vi "Test Executive.vi"(11 "Module Config":T30={"Name"="Test Executive", "Parent Q"=refnum, "Is Child?"=FALSE, "Index"=0, "Dirs"={"Root"=path "C:/MTE", "Config"=path "C:/MTE/Config", "Logs"=path "C:/MTE/Logs", "Reports"=path "C:/ATE/Reports", "App Data"=path "C:/ProgramData/Test Executive"}, "Simulate"=FALSE, "SimCtrl"=refnum}) -> ()   [LabVIEW 2018] (continued)
              tunnel: [w876] -> w869
              stop <- w876 stop-if-true
              n424 = Unbundle By Name(w880) -> ("Path"=w879:path, "Name"=w878:string)
              n425 = Equal?(x=w878, y=w877) -> (x = y?=w876:bool)
            }
            n426 = case shown="True" w869 {
              tunnel: w870 -> [_ w875]
              tunnel: [_ w874] -> _
              frame False {
              }
              frame True {
                n427 = call <vilib>:"File.Open File or Folder.vi"("Path"=w875) -> ("Error Out"=w874:errorcluster)  [unwired: 10 in]
              }
            }
          }
          frame "Config - Set Test Exec Cfg" {
            n428 = call "TestExec.Configure Test Executive Station Read and Dialog.vi"("Dialog"=TRUE, "TE Config Folder"=path "C:/MTE/Test Executive/Config" ("Path")) -> ("Changed"=w881:bool)  [unwired: 8 in, 1 out]
            n429 = case shown="True" w881 {
              frame False {
              }
              frame True {
                n430 = One Button Dialog(message="Close then relaunch Test Executive for changes to take effect.") -> ()  [unwired: 1 in, 1 out]
              }
            }
          }
          frame "Config - Set Local Station Cfg" {
            n431 = Unbundle By Name(w894) -> ("Cfg.Dirs.Config"=w889:path)
            n432 = Build Path(base path=w889, name or relative path="Local Station.ini") -> (appended path=w888:path)
            n433 = call "TestExec.Configure Local Station ID Read and Dialog.vi"("Dialog"=TRUE, "Config File"=w888) -> ("Changed"=w893:bool, "Station Out"=w890:T4)  [unwired: 8 in]
            n434 = case shown="True" w893 {
              tunnel: w891 -> [w896 w903]
              tunnel: [w896 w902] -> w892
              tunnel: w890 -> [_ w897]
              frame False {
              }
              frame True {
                n435 = Unbundle By Name(w897) -> ("Name"=w901:string, "PN"=w900:string, "SN"=w899:string, "Location"=w898:string)
                n436 = local write "Station"(w897) -> ()
                n437 = Bundle By Name(cluster=w903, "RptHdr.Station.Name"=w901, "RptHdr.Station.PN"=w900, "RptHdr.Station.SN"=w899, "RptHdr.Station.Location"=w898) -> (w902:T73)
              }
            }
          }
          frame "Config - Set File Sync" {
            w925 = T74 -5201 items=["No Error"=0, "Abort"=-2, "Misc"=-5000, "Fixture Error"=-5100, "File IO - General"=-5200, "FIle IO - Config Error"=-5201, "Instrument - General"=-5300, "Instrument - Serial Com"=-5301, "Instrument - Camera"=-5302, "Instrument - PS"=-5303, "Instrument - Oscilloscope"=-5304, "Instrument - Function Gen"=-5305, "Instrument - Load"=-5306, "Instrument - Meter"=-5307, "Instrument - Power Control"=-5308, "Instrument - Motion"=-5309, "Instrument - RF"=-5310, "System Exe"=-5400, "Image Processing"=-5500, "Communication"=-5600, "Script - Syntax Error"=-6000, "Script - Invalid Name or Param"=-6100, "Script - Timeout"=-6200, "Invalid Data"=-6300, "FW Update Error"=-6500] ("Std Code")
            # "If master was edited, copy to local"
            n438 = Variant To Data(type=FALSE, Variant=w929) -> (data=w926:bool, error out=w927:errorcluster)  [unwired: 1 in]
            n439 = flat-sequence {
              tunnel: [errorcluster {"status"=FALSE, "code"=0, "source"=""} ("error constant")] -> w920
              frame #0 {
                n440 = local write "FileSyncActive"(TRUE ("FileSyncActive")) -> ()
              }
            }
            n441 = case shown="No Error" w927 {
              tunnel: w926 -> [w958 _]
              tunnel: [w958 _] -> w915
              frame No Error {
              }
              frame Error {
              }
            }
            n442 = Unbundle By Name(w934) -> ("Cfg.Dirs.Config"=w922:path)
            n443 = Unbundle By Name(w916) -> ("Sync"=w935:refnum<class "File.Sync.lvclass">)
            n444 = Unbundle By Name(w916) -> ("CfgFilePaths.WorkingCfg"=w914:path)
            n445 = Build Path(base path=w922, name or relative path="File Sync Config.csv") -> (appended path=w910:path)
            n446 = local read "Force Sync Now"() -> (w904:bool)
            n447 = call "TestExec.Configure Select Master File Sync Config File.vi"("Dialog"=w915, "File Sync Local"=w910, "Working Config"=w914) -> ("Is Master"=w913:bool, "File Sync File"=w911:path)  [unwired: 7 in]
            n448 = call-dynamic "FileSync.Read Config.vi"("error in (no error)"=w920, "Dialog"=w915, "Config File"=w911, "File.Sync in"=w935) -> ("error out"=w919:errorcluster, "SyncItems"=w908:T14[], "Saved"=w912:bool, "File.Sync out"=w932:refnum<class "File.Sync.lvclass">)  [unwired: 4 in]
            n449 = Or(x="Enable File Sync", y=w904) -> (x .or. y?=w907:bool)
            n450 = Bundle By Name(cluster=w916, "Lists.FileSyncMaster"=w911) -> (w917:T73)
            n451 = And(x=w913, y=w912) -> (x .and. y?=w909:bool)
            n452 = case shown="True" w907 {
              tunnel: w932 -> [w937 w952]
              tunnel: [w937 w950] -> w931
              tunnel: [w938 w949] -> w930
              tunnel: w919 -> [w936 w946]
              tunnel: [w936 w942] -> w918
              tunnel: w908 -> [w938 _]
              tunnel: [_ FALSE] -> w905
              frame False {
              }
              frame True {
                n453 = control-ref of="Status"() -> (w948:refnum<vi>)
                n454 = local read "SyncType"() -> (w940:bool)
                n455 = call "String.Notification Message - Set Text Box State.vi"("error in (no error)"=w946, "Message"="Syncing Config Files, Please Wait.", "TxtBoxRef"=w948) -> ("error out"=w941:errorcluster, "OldColor"=w943:u32, "OldValue"=w944:string, "RefOut"=w945:refnum<vi>)  [unwired: 5 in]
                n456 = call-dynamic "FileSync.Update Sync.vi"("error in (no error)"=w941, "Sync Diff(F) or All(T)"=w940, "Normal(F)/Force Sync(T)"=TRUE, "File.Sync in"=w952) -> ("error out"=w942:errorcluster, "Sync Items"=w949:T14[], "File.Sync out"=w950:refnum<class "File.Sync.lvclass">)  [unwired: 3 in, 2 out]
                n457 = call "String.Notification Message - Set Text Box State.vi"("error in (no error)"=w942, "NewColor"=w943, "Message"=w944, "TxtBoxRef"=w945) -> ()  [unwired: 4 in, 4 out]
              }
            }
            "Sync Items" <- w930
            n458 = case shown="True" w909 {
              tunnel: w911 -> [_ w954]
              tunnel: w910 -> [_ w953]
              frame False {
              }
              frame True {
                n459 = call <vilib>:"File.Copy with Overwrite.vi"("Destination"=w953, "Source"=w954) -> ()  [unwired: 7 in, 3 out]
              }
            }
            n460 = flat-sequence {
              tunnel: w918 -> [_]
              frame #0 {
                n461 = local write "FileSyncActive"(FALSE ("FileSyncActive")) -> ()
              }
            }
            n462 = local write "Force Sync Now"(w905) -> ()
            n463 = Bundle By Name(cluster=w917, "Sync"=w931) -> (w933:T73)
            n464 = call "Error.Set-Change Error Info.vi"("Std Code"=w925, "error in"=w918, "Description"="Sync Files. ") -> ("error out"=w923:errorcluster)  [unwired: 8 in]
          }
          frame "Config - Set Reports" {
            w972 = T74 -5201 items=["No Error"=0, "Abort"=-2, "Misc"=-5000, "Fixture Error"=-5100, "File IO - General"=-5200, "FIle IO - Config Error"=-5201, "Instrument - General"=-5300, "Instrument - Serial Com"=-5301, "Instrument - Camera"=-5302, "Instrument - PS"=-5303, "Instrument - Oscilloscope"=-5304, "Instrument - Function Gen"=-5305, "Instrument - Load"=-5306, "Instrument - Meter"=-5307, "Instrument - Power Control"=-5308, "Instrument - Motion"=-5309, "Instrument - RF"=-5310, "System Exe"=-5400, "Image Processing"=-5500, "Communication"=-5600, "Script - Syntax Error"=-6000, "Script - Invalid Name or Param"=-6100, "Script - Timeout"=-6200, "Invalid Data"=-6300, "FW Update Error"=-6500] ("Std Code")
            n465 = Variant To Data(type=FALSE, Variant=w976) -> (data=w973:bool, error out=w974:errorcluster)  [unwired: 1 in]
            n466 = Unbundle By Name(w978) -> ("Cfg.Dirs.Config"=w966:path)
            n467 = case shown="No Error" w974 {
              tunnel: w973 -> [w979 _]
              tunnel: [w979 _] -> w964
              frame No Error {
              }
              frame Error {
              }
            }
            n468 = Unbundle By Name(w963) -> ("RptCfg"=w962:T17[])
            n469 = Build Path(base path=w966, name or relative path="Reports Config.csv") -> (appended path=w960:path)
            n470 = call "Reports.Report Config - Read.vi"("Config File"=w960, "Dialog"=w964, "Report Config In"=w962) -> ("error out"=w961:errorcluster, "Report Config Out"=w959:T17[])  [unwired: 7 in]
            "Report Config" <- w959
            n471 = Array Size(array=w959) -> (size(s)=w969:i32)
            n472 = Bundle By Name(cluster=w963, "RptCfg"=w959) -> (w977:T73)
            n473 = Initialize Array(cluster{"Open":bool} {"Open"=FALSE} ("Item"), w969) -> (w967:cluster{"Open":bool}[])
            n474 = local write "Open RprFldr"(w967) -> ()
            n475 = call "Error.Set-Change Error Info.vi"("Std Code"=w972, "error in"=w961, "Description"="Report file config.") -> ("error out"=w970:errorcluster)  [unwired: 8 in]
          }
          frame "Config - Mode Manager" {
            n476 = Unbundle By Name(w980) -> ("CfgFilePaths.ModeCfg"=w981:path)
            n477 = call "ModeMgr.Mode Setup Dialog.vi"("Mode Config File"=w981) -> ()  [unwired: 11 in]
          }
          frame "DisableResults" {
            # "DisableResults(1 or 0) \n    By default at each equence start results are enabled\n    1 == this sequence will not generate a report file\n    0 == this sequence will generate a report file"
            n478 = Variant To Data(type=string[] [], Variant=w992) -> (data=w986:string[], error out=w988:errorcluster)  [unwired: 1 in]
            n479 = Index Array(array=w986) -> (element=w985:string)  [unwired: 1 in]
            n480 = Equal?(x=w985, y="1") -> (x = y?=w983:bool)
            n481 = Bundle By Name(cluster=w990, "DisableResults"=w983) -> (w993:T73)
            n482 = case shown="Error" w988 {
              selector: w988 -> [_ w1000]
              tunnel: w987 -> [_ w997]
              tunnel: [_ w995] -> w989
              frame No Error {
              }
              frame Error {
                n483 = Format Into String(format string="Invalid Data to task %s. Expected 1D string.", w997) -> (resulting string=w996:string)  [unwired: 2 in, 1 out]
                n484 = call "Error.Set-Change Error Info.vi"("error in"=w1000, "Description"=w996, "Cust Code(0 = no change)"=-5500 ("Code(0 = no change)")) -> ("error out"=w995:errorcluster)  [unwired: 8 in]
              }
            }
          }
          frame "Get Released SW Files" {
            w1012 = T74 -5201 items=["No Error"=0, "Abort"=-2, "Misc"=-5000, "Fixture Error"=-5100, "File IO - General"=-5200, "FIle IO - Config Error"=-5201, "Instrument - General"=-5300, "Instrument - Serial Com"=-5301, "Instrument - Camera"=-5302, "Instrument - PS"=-5303, "Instrument - Oscilloscope"=-5304, "Instrument - Function Gen"=-5305, "Instrument - Load"=-5306, "Instrument - Meter"=-5307, "Instrument - Power Control"=-5308, "Instrument - Motion"=-5309, "Instrument - RF"=-5310, "System Exe"=-5400, "Image Processing"=-5500, "Communication"=-5600, "Script - Syntax Error"=-6000, "Script - Invalid Name or Param"=-6100, "Script - Timeout"=-6200, "Invalid Data"=-6300, "FW Update Error"=-6500] ("Std Code")
            n485 = for {
              N: 2 -> [_]
              tunnel: w1021 -> [w1036]
              shift-right: [w1034] -> w1023
              shift-left: _ -> [w1035]
              tunnel: w1025 -> [w1033]
              tunnel: [w1032] -> w1020 mode=indexing
              tunnel: [w1031] -> w1019
              i -> [w1037]
              stop <- w1031 stop-if-true
              n486 = case shown="1" w1037 {
                tunnel: w1036 -> [_ _]
                tunnel: [w1045 _] -> w1031
                tunnel: w1035 -> [_ w1054]
                tunnel: [w1042 w1053] -> w1034
                tunnel: w1033 -> [w1044 _]
                tunnel: [_ w1048] -> w1032
                frame 0, Default {
                  n487 = Unbundle By Name(w1044) -> ("CfgFilePaths.WorkingCfg"=w1046:path)
                  n488 = call "TestExec.Config, Get Released SW Folder Info.vi"("Station Info"=w1046) -> ("error out"=w1045:errorcluster, "Rel SW File"=w1043:path, "SW Check En"=w1039:bool, "SW Check Int(s)"=w1040:dbl)  [unwired: 5 in, 2 out]
                  n489 = Bundle By Name(cluster=T42 {"Config Folder"=path "", "Seq Folder"=path "", "Rel SW File"=path "", "SW Check Int(s)"=0.0, "Vers"=variant, "SW Check En"=FALSE}, "Rel SW File"=w1043, "SW Check Int(s)"=w1040, "Vers"=variant, "SW Check En"=w1039) -> (w1042:T42)
                }
                frame 1 {
                  n490 = Unbundle By Name(w1054) -> ("SW Check En"=w1049:bool, "Rel SW File"=w1055:path)
                  n491 = call <vilib>:"File.Check if File or Folder Exists.vi"("Path"=w1055) -> ("error out"=w1056:errorcluster, "Exists"=w1050:bool, "Dup Path"=w1057:path)  [unwired: 6 in, 2 out]
                  n492 = And(x=w1049, y=w1050) -> (x .and. y?=w1051:bool)
                  n493 = case shown="True" w1051 {
                    tunnel: w1057 -> [_ w1061]
                    tunnel: w1056 -> [_ _]
                    tunnel: [_ w1060] -> w1052
                    tunnel: [_ w1059] -> w1048
                    tunnel: [_ w1058] -> w1047
                    frame False {
                    }
                    frame True {
                      n494 = call "TestExec.Config, Get Released SW List.vi"("Path"=w1061) -> ("error out"=w1059:errorcluster, "SW List Array"=w1058:string[][], "SW List"=w1060:variant)  [unwired: 8 in]
                    }
                  }
                  "RelSWVers" <- w1047
                  n495 = Bundle By Name(cluster=w1054, "Vers"=w1052) -> (w1053:T42)
                }
              }
            }
            n496 = Unbundle By Name(w1021) -> ("Cfg.Dirs.Root"=w1017:path)
            n497 = call <vilib>:"Q.Enqueue Task.vi"("Task Name"="Maint - Scheduler", "Q In"=w1007) -> ()  [unwired: 8 in, 2 out]
            n498 = Build Path(base path=w1017, name or relative path="Config") -> (appended path=w1016:path)
            n499 = Unbundle By Name(w1023) -> ("Rel SW File"=w1001:path, "SW Check Int(s)"=w1002:dbl, "Vers"=w1022:variant, "SW Check En"=w1003:bool)
            n500 = Merge Errors(w1020, w1019) -> (w1015:errorcluster)
            n501 = case shown="False" FALSE {
              tunnel: w1016 -> [_ w1030]
              tunnel: w1015 -> [w1027 w1029]
              tunnel: [w1027 w1028] -> w1014
              frame False {
              }
              frame True {
                n502 = call "TestExec.Log SW Sync.vi"("error in (no error)"=w1029, "Folder"=w1030) -> ("error out"=w1028:errorcluster)  [unwired: 9 in]
              }
            }
            n503 = call <vilib>:"High Resolution Relative Seconds.vi"() -> ("relative seconds"=w1008:dbl)
            n504 = Bundle By Name(cluster=T12 {"Check Interval"=0.0, "SW Version List File"=path "", "Enabled"=FALSE} ("SW Check Config"), "Enabled"=w1003, "Check Interval"=w1002, "SW Version List File"=w1001) -> (→"SW Check Config":T12)
            n505 = call "Error.Set-Change Error Info.vi"("Std Code"=w1012, "Append Details"=FALSE, "error in"=w1014, "Description"="Error Reading Released SW Config File.") -> ("error out"=w1013:errorcluster)  [unwired: 7 in]
            n506 = Bundle By Name(cluster=w1025, "Health.LastVerListCk"=w1008, "CfgFilePaths.Rel_SW"=w1001, "Health.VerCkInterval"=w1002, "SW_Vers"=w1022, "Health.SW Check En"=w1003) -> (w1026:T73)
          }
          frame "Init Temp Dir" {
            n507 = Unbundle By Name(w1070) -> ("Cfg.Dirs.Root"=w1069:path)
            n508 = Build Path(base path=w1069, name or relative path="Data") -> (appended path=w1067:path)
            n509 = call <vilib>:"File.Create Folder if Does Not Exist.vi"("Path"=w1067) -> ("Dup Path"=w1065:path)  [unwired: 8 in, 2 out]
            n510 = Build Path(base path=w1065, name or relative path="Temp") -> (appended path=w1066:path)
            n511 = call <vilib>:"File.Create Folder if Does Not Exist.vi"("Path"=w1066) -> ("Dup Path"=w1063:path)  [unwired: 8 in, 2 out]
            n512 = Bundle By Name(cluster=w1062, "CfgFilePaths.DataTemp"=w1063) -> (w1071:T73)
          }
          frame "Maint - Scheduler" {
            n513 = local read "Test State"() -> (w1075:enum32{"Idle", "Running", "Completed"})
            n514 = case shown="\"Idle\", \"Completed\"" w1075 {
              tunnel: w1078 -> [w1082 w1088]
              tunnel: w1077 -> [w1080 w1086]
              tunnel: [w1082 w1085] -> w1076
              tunnel: w1074 -> [w1079 _]
              tunnel: [_ w1084] -> w1073
              tunnel: w1072 -> [_ w1083]
              frame Default {
                # "The station is not idle.\nDo nothing.\n\nMust have returned here due to the scheduled check.\nWhen test is idle again, a maint check will occurr again."
                n515 = call <vilib>:"Scheduler.AddTask.vi"("Interval(s)"=60.0, "Task Name"=w1079, "Sched Name"=w1079, "Q In"=w1080) -> ()  [unwired: 6 in, 2 out]
              }
              frame "Idle", "Completed" {
                n516 = while {
                  shift-right: [w1096] -> w1085
                  shift-left: w1088 -> [w1097]
                  shift-right: [w1094] -> _
                  shift-left: "SW" -> [w1095]
                  tunnel: w1086 -> [w1092]
                  shift-right: [w1091] -> w1084
                  shift-left: _ -> [w1090]
                  tunnel: w1083 -> [w1089]
                  stop <- w1093 stop-if-true
                  n517 = case shown="\"SW Ck\"" w1095 {
                    tunnel: w1097 -> [w1102 w1107 w1154 w1168]
                    tunnel: [w1102 w1107 w1158 w1168] -> w1096
                    tunnel: [w1101 w1105 "Done" "Done"] -> w1094
                    tunnel: [_ _ _ TRUE] -> w1093
                    tunnel: w1092 -> [_ w1110 w1160 _]
                    tunnel: [_ _ w1142 w1165] -> w1091
                    tunnel: w1090 -> [_ _ _ w1165]
                    tunnel: w1089 -> [_ _ w1148 _]
                    frame "SW" {
                      n518 = Unbundle By Name(w1102) -> ("Health.SW Check En"=w1098:bool)
                      n519 = Select(t="SW Ck", s=w1098, f="Sync") -> (s? t:f=w1101:string)
                    }
                    frame "SW Ck" {
                      n520 = Unbundle By Name(w1107) -> ("Health.VerCkInterval"=w1115:dbl)
                      n521 = Unbundle By Name(w1107) -> ("Health.LastVerListCk"=w1120:dbl)
                      n522 = Unbundle By Name(w1107) -> ("Health.LastVerCk"=w1121:dbl)
                      n523 = call <vilib>:"High Resolution Relative Seconds.vi"() -> ("relative seconds"=w1122:dbl)
                      n524 = call <vilib>:"High Resolution Relative Seconds.vi"() -> ("relative seconds"=w1119:dbl)
                      n525 = Subtract(x=w1122, y=w1121) -> (x-y=w1117:dbl)
                      n526 = Subtract(x=w1119, y=w1120) -> (x-y=w1116:dbl)
                      n527 = Subtract(x=w1115, y=w1117) -> (x-y=w1113:dbl)
                      n528 = Subtract(x=w1115, y=w1116) -> (x-y=w1111:dbl)
                      n529 = Less Or Equal To 0?(x=w1111) -> (x <= 0?=w1112:bool)
                      n530 = case shown="False" w1112 {
                        tunnel: "Get Released SW Files" -> [w1126 w1128]
                        tunnel: w1110 -> [w1125 w1129]
                        tunnel: w1111 -> [w1124 _]
                        tunnel: [w1123 w1127] -> w1109
                        frame False {
                          n531 = call <vilib>:"Scheduler.AddTask.vi"("Interval(s)"=w1124, "Task Name"=w1126, "Sched Name"=w1126, "Q In"=w1125) -> ("Q Out"=w1123:refnum<queue>)  [unwired: 6 in, 1 out]
                        }
                        frame True {
                          n532 = call <vilib>:"Q.Enqueue Task.vi"("Task Name"=w1128, "Q In"=w1129) -> ("Q Out"=w1127:refnum<queue>)  [unwired: 8 in, 1 out]
                        }
                      }
                      n533 = local read "Enable File Sync"() -> (w1103:bool)
                      n534 = Less Or Equal To 0?(x=w1113) -> (x <= 0?=w1114:bool)
                      n535 = case shown="True" w1114 {
                        tunnel: "Maint - SW Version Check" -> [w1132 w1133]
                        tunnel: w1109 -> [w1131 w1134]
                        tunnel: w1113 -> [w1130 _]
                        frame False {
                          n536 = call <vilib>:"Scheduler.AddTask.vi"("Interval(s)"=w1130, "Task Name"=w1132, "Sched Name"=w1132, "Q In"=w1131) -> ()  [unwired: 6 in, 2 out]
                        }
                        frame True {
                          n537 = call <vilib>:"Q.Enqueue Task.vi"("Task Name"=w1133, "Q In"=w1134) -> ()  [unwired: 8 in, 2 out]
                        }
                      }
                      n538 = Select(t="Sync", s=w1103, f="Done") -> (s? t:f=w1105:string)
                    }
                    frame "Sync" {
                      w1159 = "Maint - Scheduler"
                      n539 = control-ref of="Status"() -> (w1137:refnum<vi>)
                      n540 = property on="FileSyncActive" class="Bool (strict)"("Value"=TRUE ("FileSyncActive")) -> (error out=w1150:errorcluster)  [unwired: 2 in, 1 out]
                      n541 = Unbundle By Name(w1154) -> ("Sync"=w1156:refnum<class "File.Sync.lvclass">)
                      n542 = call "String.Notification Message - Set Text Box State.vi"("Message"="Syncing Config Files, Please Wait.", "TxtBoxRef"=w1137) -> ("OldColor"=w1138:u32, "OldValue"=w1139:string, "RefOut"=w1140:refnum<vi>)  [unwired: 6 in, 1 out]
                      n543 = call-dynamic "FileSync.Update Sync.vi"("error in (no error)"=w1150, "Sync Diff(F) or All(T)"="SyncType", "File.Sync in"=w1156) -> ("error out"=w1142:errorcluster, "Sync Items"=w1151:T14[], "File.Sync out"=w1155:refnum<class "File.Sync.lvclass">, "Next Sync"=w1152:dbl)  [unwired: 4 in, 1 out]
                      n544 = local write "Sync Items"(w1151) -> ()
                      n545 = case shown="Error" w1142 {
                        tunnel: ["File Sync Success" "File Sync Error"] -> w1146
                        frame No Error {
                        }
                        frame Error {
                        }
                      }
                      n546 = call "String.Notification Message - Set Text Box State.vi"("error in (no error)"=w1142, "NewColor"=w1138, "Message"=w1139, "TxtBoxRef"=w1140) -> ("error out"=w1141:errorcluster)  [unwired: 4 in, 3 out]
                      n547 = Bundle By Name(cluster=w1154, "Sync"=w1155) -> (w1153:T73)
                      n548 = Unbundle By Name(w1148) -> ("Log"=w1147:refnum<class "Event Notification.lvclass">)
                      n549 = flat-sequence {
                        tunnel: w1141 -> [_]
                        frame #0 {
                          n550 = property on="FileSyncActive" class="Bool (strict)"("Value"=FALSE ("FileSyncActive")) -> ()  [unwired: 2 in, 2 out]
                        }
                      }
                      n551 = Bundle By Name(cluster=w1153, "Health.Init"=FALSE) -> (w1158:T73)
                      n552 = call <vilib>:"Scheduler.AddTask.vi"("Interval(s)"=w1152, "Task Name"=w1159, "Sched Name"=w1159, "Q In"=w1160) -> ()  [unwired: 6 in, 2 out]
                      n553 = call <vilib>:"Event Notification.Status Message.vi"("Display"=FALSE, "Log"=TRUE, "Level"=Event_Log.Log_Level."Verbose", "Message"=w1146, "Event Notification in"=w1147) -> ()  [unwired: 7 in]
                    }
                    frame "Done", Default {
                    }
                  }
                }
              }
            }
          }
          frame "Maint - SW Version Check" {
            # "TODO: \nAt launch:\n  Need to get version from Sta\n  Get version of all seq and limit at init"
            n554 = Unbundle By Name(w1175) -> ("SW_Vers"=w1177:variant, "RptHdr.Station.SW_Config.SW_Item"=w1178:T31[])  [unwired: 1 out]
            n555 = call <vilib>:"High Resolution Relative Seconds.vi"() -> ("relative seconds"=w1176:dbl)
            n556 = Get Date/Time In Seconds() -> (seconds since 1Jan1904=→"LastVerCkTime":timestamp)
            n557 = Bundle By Name(cluster=w1175, "Health.LastVerCk"=w1176) -> (w1174:T73)
            n558 = call <vilib>:"Q.Enqueue Task.vi"("Task Name"="Maint - Scheduler", "Q In"=w1172) -> ("Q Out"=w1171:refnum<queue>)  [unwired: 8 in, 1 out]
            n559 = for {
              tunnel: w1178 -> [w1190] mode=indexing
              tunnel: w1177 -> [w1191]
              tunnel: w1171 -> [w1188]
              tunnel: [w1184] -> w1169 mode=indexing
              n560 = Unbundle By Name(w1190) -> ("Name"=w1185:string, "PN"=w1182:string, "Version"=w1183:string)
              n561 = Get Variant Attribute(Variant=w1191, name=w1185, default value (empty Variant)="") -> (found=w1180:bool, value=w1186:string)  [unwired: 1 in, 2 out]
              n562 = Not Equal?(x=w1183, y=w1186) -> (x != y?=w1187:bool)
              n563 = And(x=w1180, y=w1187) -> (x .and. y?=w1181:bool)
              n564 = Bundle("Name"=w1185, "PN"=w1182, "Version"=w1183, w1180, w1181) -> (w1184:T75)  [unwired: 1 in]
              n565 = case shown="True" w1181 {
                tunnel: w1188 -> [_ w1200]
                tunnel: w1185 -> [_ w1193]
                tunnel: w1186 -> [_ w1196]
                tunnel: w1183 -> [_ w1194]
                frame False {
                }
                frame True {
                  n566 = Format Into String(format string="SW '%s' is not the released version.  Local ver is '%s' and released ver is '%s'.", w1193, w1194, w1196) -> (resulting string=w1195:string)  [unwired: 2 in, 1 out]
                  n567 = Bundle By Name(cluster=errorcluster {"status"=TRUE, "code"=7000, "source"=""} ("error constant"), "source"=w1195) -> (w1198:errorcluster)
                  n568 = To Variant(anything=TestExec.Health_State_Command."Set Warning" ("Health State Cmd")) -> (Variant=w1204:variant)
                  n569 = To Variant(anything=w1198) -> (Variant=w1201:variant)
                  n570 = call <vilib>:"Q.Enqueue App.vi"("Data2"=w1201, "Top of Q"=TRUE, "Data1"=w1204, "Task Name"="Health Status", "Q In"=w1200) -> ()  [unwired: 5 in, 2 out]
                }
              }
            }
            "Station SW Versions" <- w1169
          }
          frame "Operator - Create Report" {
            # "TODO - Create Report"
            n571 = Unbundle By Name(w1205) -> ()  [unwired: 1 out]
          }
          frame "Operator - Operator Change" {
            n572 = local read "Test Ctrl Tab"() -> (w1211:enum32{"Idle", "Running", "Completed"})
            n573 = call <vilib>:"Trim Whitespace.vi"("string"="Operator") -> ("trimmed string"=w1207:string)  [unwired: 1 in]
            n574 = Bundle By Name(cluster=w1210, "RptHdr.Test Run.Operator"=w1207) -> (w1209:T73)
            n575 = local write "Operator"(w1207) -> ()
            n576 = case shown="\"Idle\"" w1211 {
              tunnel: w1212 -> [_ w1214]
              frame Default {
              }
              frame "Idle" {
                n577 = To Variant(anything="Operator Change" ("Task Name")) -> (Variant=w1216:variant)
                n578 = call <vilib>:"Q.Enqueue Seq.vi"("Data1"=w1216, "Seq Task Name"="Test Idle" ("Task Name"), "Q In"=w1214) -> ()  [unwired: 7 in, 2 out]
              }
            }
          }
          frame "Operator - Set Mode" {
            n579 = Variant To Data(type=FALSE, Variant=w1222) -> (data=w1219:bool, error out=w1220:errorcluster)  [unwired: 1 in]
            n580 = Unbundle By Name(w1231) -> ("ModeMgr"=w1230:refnum<class "Mode Manager.lvclass">)
            n581 = case shown="No Error" w1220 {
              tunnel: w1219 -> [w1232 _]
              tunnel: [w1232 FALSE] -> w1218
              frame No Error {
              }
              frame Error {
              }
            }
            n582 = call "ModeMgr.Set Mode.vi"("Init"=w1218, "ModeMgr In"=w1230) -> ("Settings"=w1225:T76[], "Mode"=w1226:string, "ModeMgr Out"=w1229:refnum<class "Mode Manager.lvclass">, "Changed"=w1223:bool)  [unwired: 5 in, 1 out]
            n583 = case shown="True" w1223 {
              tunnel: w1231 -> [w1234 w1242]
              tunnel: w1229 -> [_ w1248]
              tunnel: [w1234 w1247] -> w1228
              tunnel: w1226 -> [_ w1241]
              tunnel: w1225 -> [_ w1246]
              tunnel: w1224 -> [_ w1244]
              frame False {
              }
              frame True {
                n584 = Unbundle By Name(w1242) -> ("Lists.DisableRouteCk"=w1238:bool)
                n585 = call <vilib>:"Q.Enqueue Task.vi"("Task Name"="Options - Set", "Q In"=w1244) -> ("Q Out"=w1236:refnum<queue>)  [unwired: 8 in, 1 out]
                n586 = call "TestExec.Set Option Controls.vi"("Disable SN Route Ck"=w1238, "TE Opts"=w1246, "TE Opts In"=T20 {"DispDetails"=FALSE, "NotResetSN"=FALSE, "NotValOper"=FALSE, "NotValSN"=FALSE, "DisResults"=FALSE, "StaModule"=FALSE, "EditEQ"=FALSE, "ClrWarn"=FALSE, "ClrErr"=FALSE, "ViewCfg"=FALSE, "SetOpts"=FALSE, "ContOnErr"=FALSE, "ContOnFail"=FALSE, "DisMetrics"=FALSE, "SelSeq"=FALSE, "GenRpt"=FALSE, "DisStartWithSN"=FALSE, "Auto Repeat Seq En"=FALSE, "DataDirEn"=FALSE, "SNRouteCk"=FALSE} ("Opts")) -> ("TE Opts Out"=w1239:T20)  [unwired: 8 in]
                n587 = call <vilib>:"Q.Enqueue Seq.vi"("Seq Task Name"="Test Reset", "Q In"=w1236) -> ()  [unwired: 8 in, 2 out]
                n588 = Unbundle By Name(w1239) -> ("SNRouteCk"=w1237:bool)
                n589 = Equal?(x=w1241, y="Production") -> ()  [unwired: 1 out]
                n590 = local write "TE Opts"(w1239) -> ()
                n591 = Bundle By Name(cluster=w1242, "ModeMgr"=w1248, "RptHdr.Test Run.Mode"=w1241, "Opts"=w1239) -> (w1247:T73)
                n592 = local write "Route Check"(w1237) -> ()
              }
            }
          }
          frame "Operator - Set Result EN" {
            n593 = control-ref of="Result Sel"() -> (w1249:refnum<vi>)
            n594 = Greater Than 0?(x="ReportEn") -> (x > 0?=w1250:bool)
            n595 = call "TestExec.Result Option, Set Enable_Disabel Color.vi"("Result Sel"=w1249) -> ()  [unwired: 11 in]
            n596 = Bundle By Name(cluster=w1255, "Opts.DisResults"=w1250) -> (w1254:T73)
            n597 = local read "TE Opts"() -> (w1253:T20)
            n598 = Bundle By Name(cluster=w1253, "DisResults"=w1250) -> (w1252:T20)
            n599 = local write "TE Opts"(w1252) -> ()
          }
          frame "Operator - SN Change" {
            n600 = local read "Test Ctrl Tab"() -> (w1261:enum32{"Idle", "Running", "Completed"})
            n601 = call <vilib>:"Trim Whitespace.vi"("string"="SN") -> ("trimmed string"=w1257:string)  [unwired: 1 in]
            n602 = local write "SN"(w1257) -> ()
            n603 = Bundle By Name(cluster=w1260, "RptUUT.UUTInfo.SN"=w1257) -> (w1259:T73)
            n604 = case shown="\"Idle\"" w1261 {
              tunnel: w1262 -> [_ w1265]
              frame Default {
              }
              frame "Idle" {
                n605 = To Variant(anything="SN Change") -> (Variant=w1267:variant)
                n606 = call <vilib>:"Q.Enqueue Seq.vi"("Data1"=w1267, "Seq Task Name"="Test Idle" ("Task Name"), "Q In"=w1265) -> ()  [unwired: 7 in, 2 out]
              }
            }
          }
          frame "Operator Comment" {
            w1275 = T39 0 items=["LOG", "PASS", "FAIL", "ERROR"] ("Status")
            w1277 = "Comment"
            n607 = Variant To Data(type="", Variant=w1281) -> (data=w1276:string)  [unwired: 1 in, 1 out]
            n608 = Bundle By Name(cluster=T43 {"Cnt"=0, "Step"="", "Category"="", "Name"="", "Value"="", "Status"=0, "Code"=0, "Desc"="", "Time"=timestamp(0 s since 1904-01-01)} ("Attribute"), "Category"=w1277, "Name"=w1277, "Value"=w1276, "Status"=w1275, "Code"=0, "Desc"="") -> (w1272:T43)
            n609 = Build Array(w1272) -> (w1271:T43[])
            n610 = To Variant(anything=w1271) -> (Variant=w1270:variant)
            n611 = call <vilib>:"Q.Enqueue Task.vi"("Data1"=w1270, "Task Name"="Result - Attributes" ("Desc"), "Q In"=w1268) -> ()  [unwired: 7 in, 2 out]
          }
          frame "Operator YesNo Input" {
            n612 = Variant To Data(type=FALSE, Variant=w1295) -> (data=w1287:bool)  [unwired: 1 in, 1 out]
            n613 = Select(t="Yes", s=w1287, f="No") -> (s? t:f=w1284:string)
            n614 = Unbundle By Name(w1293) -> ("SeqMgr"=w1290:refnum<class "SeqMgr.lvclass">)
            n615 = Build Array("Operator_YesNo_Input", w1284) -> (w1289:string[])
            n616 = Build Array(w1289) -> (w1283:string[][])
            n617 = call <vilib>:"SeqMgr.Variables - Add, Replace.vi"("Name, Value"=w1283, "SeqMgr in"=w1290) -> ("SeqMgr out"=w1291:refnum<class "SeqMgr.lvclass">)  [unwired: 8 in, 1 out]
            n618 = Bundle By Name(cluster=w1293, "SeqMgr"=w1291) -> (w1292:T73)
          }
          frame "Result Comment" {
            n619 = local read "Start Time"() -> (w1299:timestamp)
            n620 = Unbundle By Name(w1304) -> ("RptHdr.Test Run.Comment"=w1321:string)
            n621 = local read "Comment At End"() -> (w1319:bool)
            n622 = Unbundle By Name(w1304) -> ("SeqMgr"=w1305:refnum<class "SeqMgr.lvclass">)
            n623 = Unbundle By Name(w1304) -> ("Lists.CmtPrmpt"=w1320:bool)
            n624 = call <vilib>:"SeqMgr.Variables - Get.vi"("SeqMgr in"=w1305) -> ("Vars"=w1303:variant)  [unwired: 8 in, 2 out]
            n625 = Format Date/Time String(time format string (%c)="%Y%m%d_%H%M%S", seconds (now)=w1299) -> (date/time string=w1297:string)  [unwired: 1 in]
            n626 = call <vilib>:"SeqMgr.Variables, Populate Variable Value Including Array Indices.vi"("String"="UUTDir", "Variables"=w1303) -> ("error out"=w1302:errorcluster, "String Out"=w1298:string)  [unwired: 7 in, 1 out]
            n627 = case shown="False" w1320 {
              tunnel: w1321 -> [_ w1329]
              tunnel: [w1325 w1329] -> w1313
              tunnel: w1319 -> [w1324 _]
              tunnel: "Comment" -> [w1323 _]
              frame False {
                n628 = case shown="False" w1324 {
                  tunnel: [w1326 w1328] -> w1325
                  tunnel: w1323 -> [w1326 w1327]
                  frame False {
                  }
                  frame True {
                    n629 = call "TestExec.Prompt for entering Comment.vi"("Comment"=w1327) -> ("Comment Out"=w1328:string)  [unwired: 10 in]
                  }
                }
              }
              frame True {
                # "Already entered comment"
              }
            }
            n630 = Unbundle By Name(w1306) -> ("Log"=w1310:refnum<class "Event Notification.lvclass">)
            n631 = call <vilib>:"Clear Errors.vi"("error in (no error)"=w1302) -> ()  [unwired: 5 in, 2 out]
            n632 = Format Into String(format string="Test End.  Start Time = \"%s\", UUTDir = \"%s\"", w1297, w1298) -> (resulting string=w1311:string)  [unwired: 2 in, 1 out]
            n633 = call <vilib>:"Event Notification.Status Message.vi"("Log"=TRUE, "Level"=Event_Log.Log_Level."Debug1", "Message"=w1311, "Event Notification in"=w1310) -> ()  [unwired: 8 in]
            n634 = case shown="False" "PersistCmt" {
              tunnel: w1313 -> [_ _]
              frame False {
                n635 = invoke on="Comment" class="Str" method="Reinit To Default"() -> ()  [unwired: 3 in, 3 out]
              }
              frame True {
              }
            }
            n636 = call <vilib>:"Search and Replace Pattern.vi"("string"=w1313, "regular expression (\"\")"="\n", "replace string (\"\")"="| " ("regular expression (\"\")"), "replace all? (F)"=TRUE) -> ("result string"=w1317:string)  [unwired: 1 in, 1 out]
            n637 = Bundle By Name(cluster=w1304, "RptHdr.Test Run.Comment"=w1317) -> (w1322:T73)
          }
          frame "Options - Set" {
            n638 = Bundle By Name(cluster=w1332, "Opts"="TE Opts") -> (w1330:T73)
            n639 = while {
              tunnel: "TE Opts" -> [w1339]
              tunnel: w1333 -> [w1338]
              tunnel: w1332 -> [w1337]
              shift-right: [w1335] -> w1331
              shift-left: w1330 -> [w1336]
              i -> [w1340]
              stop <- w1341 stop-if-true
              n640 = case shown="13" w1340 {
                tunnel: [_ _ _ _ _ _ _ _ _ _ _ _ _ _ TRUE] -> w1341
                tunnel: w1339 -> [w1345 w1359 w1366 w1372 w1378 w1393 w1408 w1424 w1433 w1440 w1447 w1458 w1473 _ _]
                tunnel: w1338 -> [_ w1352 _ _ _ w1389 w1406 _ _ _ _ _ w1469 _ _]
                tunnel: w1337 -> [_ _ _ _ _ w1384 w1403 w1421 _ _ _ w1463 _ w1480 _]
                tunnel: [_ _ _ _ _ _ w1399 _ _ _ _ _ w1467 _ _] -> _
                tunnel: w1336 -> [w1342 w1348 w1363 w1369 w1375 w1381 w1394 w1418 w1431 w1436 w1445 w1455 w1466 w1481 w1487]
                tunnel: [w1342 w1348 w1363 w1369 w1375 w1381 w1394 w1419 w1431 w1436 w1445 w1455 w1466 w1481 w1487] -> w1335
                frame 0 {
                  n641 = Unbundle By Name(w1345) -> ("DispDetails"=w1343:bool)
                  n642 = property on="Test Status Tab" class="TabCtl (strict)"("Tabs Visible?"=w1343) -> (error out=w1344:errorcluster)  [unwired: 2 in, 1 out]
                  n643 = property on="Image Path" class="Path"("Visible"=w1343) -> ()  [unwired: 2 in, 2 out]
                  n644 = case shown="False" w1343 {
                    tunnel: w1344 -> [w1347 _]
                    frame False {
                      n645 = property on="Test Status Tab" class="TabCtl (strict)"(error in=w1347, "Value"=0) -> ()  [unwired: 1 in, 2 out]
                    }
                    frame True {
                    }
                  }
                }
                frame 1 {
                  w1353 = "Show Station Module"
                  n646 = Unbundle By Name(w1359) -> ("StaModule"=w1351:bool)
                  n647 = case shown="False" w1351 {
                    tunnel: [_ TRUE] -> w1350
                    tunnel: [T36."Disabled and Grayed Out" ("Disabled") T36."Enabled" ("Disabled")] -> w1349
                    frame False {
                    }
                    frame True {
                    }
                  }
                  n648 = Unbundle By Name(w1352) -> ("Menu Ref"=w1358:refnum<k9>)
                  n649 = Get Menu Item Info(7:w1353, 11:w1358) -> (0:w1355:errorcluster, 2:w1356:string, 3:w1357:refnum<k9>)  [unwired: 1 in, 4 out]
                  n650 = property on="Show Station Module" class="Bool"("DisabledEnum"=w1349) -> ()  [unwired: 2 in, 2 out]
                  n651 = Set Menu Item Info(7:w1353, 8:w1355, 9:w1350, 10:w1356, 11:w1357) -> (0:w1354:errorcluster)  [unwired: 2 in, 1 out]
                  n652 = call <vilib>:"Clear Errors.vi"("error in (no error)"=w1354) -> ()  [unwired: 5 in, 2 out]
                }
                frame 2 {
                  n653 = Unbundle By Name(w1366) -> ("EditEQ"=w1365:bool)
                  n654 = case shown="False" w1365 {
                    tunnel: [T36."Disabled" ("Disabled") T36."Enabled" ("Disabled")] -> w1364
                    frame False {
                    }
                    frame True {
                    }
                  }
                  n655 = property on="Equipment List" class="Tbl (strict)"("DisabledEnum"=w1364) -> ()  [unwired: 2 in, 2 out]
                }
                frame 3 {
                  n656 = Unbundle By Name(w1372) -> ("ClrWarn"=w1371:bool)
                  n657 = case shown="False" w1371 {
                    tunnel: [T36."Disabled and Grayed Out" ("Disabled") T36."Enabled" ("Disabled")] -> w1370
                    frame False {
                    }
                    frame True {
                    }
                  }
                  n658 = property on="Clear Warnings" class="Bool"("DisabledEnum"=w1370) -> ()  [unwired: 2 in, 2 out]
                }
                frame 4 {
                  n659 = Unbundle By Name(w1378) -> ("ClrErr"=w1377:bool)
                  n660 = case shown="False" w1377 {
                    tunnel: [T36."Disabled and Grayed Out" ("Disabled") T36."Enabled" ("Disabled")] -> w1376
                    frame False {
                    }
                    frame True {
                    }
                  }
                  n661 = property on="Clear Errors" class="Bool"("DisabledEnum"=w1376) -> ()  [unwired: 2 in, 2 out]
                  n662 = property on="Clear Errors and Warnings" class="Bool"("DisabledEnum"=w1376) -> ()  [unwired: 2 in, 2 out]
                  n663 = property on="Test Metrics Reset" class="Bool"("DisabledEnum"=w1376) -> ()  [unwired: 2 in, 2 out]
                  n664 = property on="Test Cycle Cnt Reset" class="Bool"("DisabledEnum"=w1376) -> ()  [unwired: 2 in, 2 out]
                }
                frame 5 {
                  w1390 = "Config" ("menu tag")
                  n665 = Unbundle By Name(w1384) -> ("RptHdr.Test Run.Mode"=w1387:string)
                  n666 = Unbundle By Name(w1393) -> ("ViewCfg"=w1383:bool)
                  n667 = Equal?(x=w1387, y="Engineering") -> (x = y?=w1385:bool)
                  n668 = Or(x=w1383, y=w1385) -> (x .or. y?=w1382:bool)
                  n669 = control-ref of="Funct Tab"() -> (w1392:refnum<vi>)
                  n670 = Unbundle By Name(w1389) -> ("Menu Ref"=w1388:refnum<k9>)
                  n671 = call <vilib>:"CtrlUtil.ShowHide Tab Page.vi"("Show"=w1382, "Tab Name"="Config", "Tab Control"=w1392) -> ()  [unwired: 2 in]
                  n672 = Set Menu Item Info(7:w1390, 9:w1382, 10:w1390, 11:w1388) -> ()  [unwired: 3 in, 2 out]
                }
                frame 6 {
                  n673 = Unbundle By Name(w1403) -> ("RptHdr.Test Run.Mode"=w1405:string)
                  n674 = Unbundle By Name(w1408) -> ("SetOpts"=w1401:bool)
                  n675 = Unbundle By Name(w1406) -> ("Menu Ref"=w1395:refnum<k9>)
                  n676 = Equal?(x=w1405, y="Engineering") -> (x = y?=w1402:bool)
                  n677 = Or(x=w1401, y=w1402) -> (x .or. y?=w1400:bool)
                  n678 = case shown="False" w1400 {
                    tunnel: [T36."Disabled and Grayed Out" ("Disabled") w1416] -> w1398
                    tunnel: [T36."Disabled" ("Disabled") w1416] -> w1407
                    tunnel: [_ TRUE] -> w1397
                    frame False {
                    }
                    frame True {
                      w1416 = T36."Enabled" ("Disabled")
                    }
                  }
                  n679 = property on="Configure Reports" class="Bool"("DisabledEnum"=w1398) -> ()  [unwired: 2 in, 2 out]
                  n680 = property on="Open SW Version File" class="Bool"("DisabledEnum"=w1398) -> ()  [unwired: 2 in, 2 out]
                  n681 = for {
                    tunnel: [w1412] -> w1399
                    tunnel: w1397 -> [w1411]
                    tunnel: string[] ["Test Executive", "Local Station", "File Sync", "Test Reports", "Mode Manager", "Config_Config Folder", "Config_Test Sequence Folder"] -> [w1410] mode=indexing
                    tunnel: w1395 -> [w1409]
                    n682 = call <vilib>:"Menu.Enable Item.vi"("Enable"=w1411, "Tag"=w1410, "Menu Ref"=w1409) -> ("error out"=w1412:errorcluster)  [unwired: 7 in, 1 out]
                  }
                  n683 = property on="Result Sel" class="Ring (strict)"("DisabledEnum"=w1407) -> ()  [unwired: 2 in, 2 out]
                  n684 = property on="TE Opts" class="Clust (strict)"("DisabledEnum"=w1398) -> ()  [unwired: 2 in, 2 out]
                }
                frame 7 {
                  n685 = Unbundle By Name(w1421) -> ("Lists.Default Seq"=w1420:i32)
                  n686 = Unbundle By Name(w1424) -> ("SelSeq"=w1423:bool)
                  n687 = case shown="False" w1423 {
                    tunnel: [T36."Disabled" ("Disabled") T36."Enabled" ("Disabled")] -> w1417
                    tunnel: [u32 0 u32 16860] -> w1422
                    tunnel: w1420 -> [w1425 _]
                    frame False {
                      n688 = To Unsigned Word Integer(number=w1425) -> (unsigned 16bit integer=w1426:u16)
                      n689 = property on="Sequence" class="Ring (strict)"("Value"=w1426) -> ()  [unwired: 2 in, 2 out]
                    }
                    frame True {
                    }
                  }
                  n690 = property on="Sequence" class="Ring (strict)"("DisabledEnum"=w1417, "RingText.TextColor"=w1422) -> ()  [unwired: 2 in, 2 out]
                  n691 = Bundle By Name(cluster=w1418, "PreTestCk.SeqEn"=w1417) -> (w1419:T73)
                }
                frame 8 {
                  n692 = Unbundle By Name(w1433) -> ("GenRpt"=w1432:bool)
                  n693 = case shown="False" w1432 {
                    tunnel: [T36."Disabled and Grayed Out" ("Disabled") T36."Enabled" ("Disabled")] -> _
                    frame False {
                    }
                    frame True {
                    }
                  }
                }
                frame 9 {
                  n694 = Unbundle By Name(w1440) -> ("DisStartWithSN"=w1439:bool)
                  n695 = case shown="True" w1439 {
                    tunnel: [T36."Disabled and Grayed Out" ("Disabled") T36."Enabled" ("Disabled")] -> w1438
                    tunnel: [TRUE w1443] -> w1437
                    frame False {
                    }
                    frame True {
                      n696 = local read "Start with SN Entry"() -> (w1443:bool)
                    }
                  }
                  n697 = local write "Start with SN Entry"(w1437) -> ()
                  n698 = property on="Start with SN Entry" class="Bool (strict)"("DisabledEnum"=w1438) -> ()  [unwired: 2 in, 2 out]
                }
                frame 10 {
                  n699 = Unbundle By Name(w1447) -> ("DisResults"=w1446:bool)
                  n700 = flat-sequence {
                    tunnel: w1446 -> [w1449]
                    frame #0 {
                      n701 = case shown="False" w1449 {
                        tunnel: [w1450 w1451] -> w1448
                        frame False {
                          w1450 = T8 0 items=["Enabled", "Disabled"] ("Result Sel")
                        }
                        frame True {
                          w1451 = T8 1 items=["Enabled", "Disabled"] ("Result Sel")
                        }
                      }
                      n702 = local write "ReportEn"(w1448) -> ()
                    }
                    frame #1 {
                      n703 = control-ref of="Result Sel"() -> (w1452:refnum<vi>)
                      n704 = call "TestExec.Result Option, Set Enable_Disabel Color.vi"("Result Sel"=w1452) -> ()  [unwired: 11 in]
                    }
                  }
                }
                frame 11 {
                  n705 = Unbundle By Name(w1463) -> ("RptHdr.Test Run.Mode"=w1460:string)
                  n706 = Unbundle By Name(w1458) -> ("Auto Repeat Seq En"=w1457:bool)
                  n707 = Equal?(x=w1460, y="Engineering") -> (x = y?=w1453:bool)
                  n708 = Or(x=w1457, y=w1453) -> (x .or. y?=w1456:bool)
                  n709 = Not(x=w1453) -> (.not. x?=w1454:bool)
                  n710 = case shown="True" w1456 {
                    tunnel: [TRUE ("Repeat Seq") FALSE ("Repeat Seq")] -> w1462
                    frame True {
                    }
                    frame False {
                    }
                  }
                  n711 = local write "Enable File Sync"(w1454) -> ()
                  n712 = local write "Repeat Seq"(FALSE ("Repeat Seq")) -> ()
                  n713 = property on="Repeat Seq" class="Bool (strict)"("Visible"=w1462) -> ()  [unwired: 2 in, 2 out]
                  n714 = property on="RepeatInt(s)" class="DigNum (strict)"("Visible"=w1462) -> ()  [unwired: 2 in, 2 out]
                }
                frame 12 {
                  # "Make always enabled"
                  n715 = Unbundle By Name(w1473) -> ("DataDirEn"=w1472:bool)
                  n716 = Unbundle By Name(w1469) -> ("Menu Ref"=w1468:refnum<k9>)
                  n717 = case shown="False" w1472 {
                    tunnel: [TRUE TRUE] -> w1470
                    frame False {
                    }
                    frame True {
                    }
                  }
                  n718 = call <vilib>:"Menu.Enable Item.vi"("Enable"=w1470, "Tag"="Data", "Menu Ref"=w1468) -> ("error out"=w1467:errorcluster)  [unwired: 7 in, 1 out]
                }
                frame 13 {
                  n719 = Unbundle By Name(w1480) -> ("RptHdr.Test Run.Mode"=w1479:string)
                  n720 = case shown="Default" w1479 {
                    tunnel: [T36."Enabled" ("Disabled") T36."Disabled and Grayed Out" ("Disabled")] -> w1477
                    tunnel: [w1483 w1485] -> w1478
                    tunnel: [w1482 w1485] -> w1476
                    frame Default {
                      n721 = property on="Comment At End" class="Bool (strict)"() -> ("Value"=w1483:bool)  [unwired: 2 in, 2 out]
                      n722 = property on="PersistCmt" class="Bool (strict)"() -> ("Value"=w1482:bool)  [unwired: 2 in, 2 out]
                    }
                    frame "Production" {
                      w1485 = FALSE
                    }
                  }
                  n723 = property on="Comment At End" class="Bool (strict)"("DisabledEnum"=w1477, "Value"=w1478) -> ()  [unwired: 2 in, 2 out]
                  n724 = property on="PersistCmt" class="Bool (strict)"("DisabledEnum"=w1477, "Value"=w1476) -> ()  [unwired: 2 in, 2 out]
                }
                frame Default {
                }
              }
            }
          }
          frame "PLC - Enable" {
            n725 = property on="PLC" class="Bool (strict)"() -> ("Visible"=w1489:bool)  [unwired: 2 in, 2 out]
            n726 = case shown="True" w1489 {
              frame False {
              }
              frame True {
                n727 = To Variant(anything="PLC Enable") -> (Variant=w1493:variant)
                n728 = call <vilib>:"Q.Enqueue Task.vi"("Data1"=w1493, "Q Name"="PLC", "Task Name"="TE Enable PLC") -> ()  [unwired: 7 in, 2 out]
              }
            }
          }
          frame "PLC - Running Done" {
            n729 = Unbundle By Name(w1501) -> ("Subscr"=w1500:T58[])
            n730 = for {
              tunnel: w1500 -> [w1505] mode=indexing
              tunnel: w1499 -> [w1504]
              tunnel: [w1506] -> w1498
              tunnel: [w1505] -> w1497 mode=indexing
              tunnel: [w1504] -> w1496
              stop <- w1506 stop-if-true
              n731 = Unbundle By Name(w1505) -> ("Name"=w1507:string)
              n732 = Equal?(x=w1507, y=w1504) -> (x = y?=w1506:bool)
            }
            n733 = case shown="True" w1498 {
              tunnel: w1501 -> [_ w1511]
              tunnel: w1497 -> [_ _]
              tunnel: w1496 -> [_ w1510]
              frame False {
              }
              frame True {
                n734 = Unbundle By Name(w1511) -> ("StaApp"=w1512:string)
                n735 = To Variant(anything=FALSE) -> (Variant=w1508:variant)
                n736 = call <vilib>:"Q.Enqueue Task.vi"("Data1"=w1508, "Q Name"=w1512, "Task Name"=w1510) -> ()  [unwired: 7 in, 2 out]
              }
            }
            n737 = local write "PLC Running"(FALSE ("PLC Running")) -> ()
          }
          frame "PLC - Running Start" {
            n738 = Unbundle By Name(w1518) -> ("Subscr"=w1517:T58[])
            n739 = for {
              tunnel: w1517 -> [w1522] mode=indexing
              tunnel: w1516 -> [w1521]
              tunnel: [w1523] -> w1515
              tunnel: [w1522] -> w1514 mode=indexing
              tunnel: [w1521] -> w1513
              stop <- w1523 stop-if-true
              n740 = Unbundle By Name(w1522) -> ("Name"=w1524:string)
              n741 = Equal?(x=w1524, y=w1521) -> (x = y?=w1523:bool)
            }
            n742 = case shown="True" w1515 {
              tunnel: w1518 -> [_ w1528]
              tunnel: w1514 -> [_ _]
              tunnel: w1513 -> [_ w1527]
              frame False {
              }
              frame True {
                n743 = Unbundle By Name(w1528) -> ("StaApp"=w1529:string)
                n744 = To Variant(anything=TRUE) -> (Variant=w1525:variant)
                n745 = call <vilib>:"Q.Enqueue Task.vi"("Data1"=w1525, "Q Name"=w1529, "Task Name"=w1527) -> ()  [unwired: 7 in, 2 out]
              }
            }
            n746 = local write "PLC Running"(TRUE ("PLC Running")) -> ()
          }
          frame "PLC - Set Start" {
            n747 = property on="PLC" class="Bool (strict)"() -> ("Visible"=w1533:bool)  [unwired: 2 in, 2 out]
            n748 = case shown="True" w1533 {
              frame False {
              }
              frame True {
                n749 = call <vilib>:"Q.Enqueue Task.vi"("Q Name"="PLC", "Task Name"="PLC - Set Start") -> ()  [unwired: 8 in, 2 out]
              }
            }
            n750 = call <vilib>:"Q.Enqueue Task.vi"("Q Name"="Wiggler", "Task Name"="Test Start") -> ()  [unwired: 8 in, 2 out]
          }
          frame "PLC - Show State" {
            n751 = property on="PLC" class="Bool (strict)"() -> ("Visible"=w1537:bool)  [unwired: 2 in, 2 out]
            n752 = case shown="True" w1537 {
              frame False {
              }
              frame True {
                n753 = call <vilib>:"Q.Enqueue Task.vi"("Q Name"="PLC", "Task Name"="Show Panel") -> ()  [unwired: 8 in, 2 out]
              }
            }
          }
          frame "Read Limits" {
            n754 = while {
              tunnel: w1547 -> [w1560]
              tunnel: [w1559] -> w1553
              tunnel: w1546 -> [w1556]
              tunnel: [w1555] -> w1543
              i -> [w1558]
              stop <- w1557 stop-if-true
              n755 = case shown="0, Default" w1558 {
                tunnel: w1560 -> [w1568 _ w1582]
                tunnel: [w1564 _ w1576] -> w1559
                tunnel: [w1561 TRUE w1574] -> w1557
                tunnel: w1556 -> [_ _ w1581]
                tunnel: [w1563 w1569 w1575] -> w1555
                frame 1 {
                  n756 = Unbundle By Name(w1568) -> ("Cfg.Dirs.Config"=w1567:path)
                  n757 = Build Path(base path=w1567, name or relative path="Limits") -> (appended path=w1565:path)
                  n758 = call "TestExec.Get Limit File.vi"("Folder"=w1565) -> ("error out"=w1563:errorcluster, "Path"=w1564:path)  [unwired: 7 in, 2 out]
                  n759 = Unbundle By Name(w1563) -> ("status"=w1562:bool)
                  n760 = Not(x=w1562) -> (.not. x?=w1561:bool)
                }
                frame 2 {
                  # "No Limits Found"
                  n761 = call "Error.Set-Change Error Info.vi"("Description"="Test Limit File Not Found", "Cust Code(0 = no change)"=-5200 ("Code(0 = no change)"), "Set Error"=TRUE) -> ("error out"=w1569:errorcluster)  [unwired: 8 in]
                }
                frame 0, Default {
                  n762 = Unbundle By Name(w1581) -> ("RptHdr.Test Sequence.Name"=w1580:string)
                  n763 = Unbundle By Name(w1582) -> ("Cfg.Dirs.Root"=w1584:path)
                  n764 = Build Path(base path=w1584, name or relative path="Sequences" ("section")) -> (appended path=w1579:path)
                  n765 = Build Path(base path=w1579, name or relative path=w1580) -> (appended path=w1577:path)
                  n766 = call "TestExec.Get Limit File.vi"("Folder"=w1577) -> ("error out"=w1575:errorcluster, "Path"=w1576:path)  [unwired: 7 in, 2 out]
                  n767 = Unbundle By Name(w1575) -> ("status"=w1578:bool)
                  n768 = Not(x=w1578) -> (.not. x?=w1574:bool)
                }
              }
            }
            n769 = call "Result.Load Test Limits from XML File.vi"("error in (no error)"=w1543, "Limit File Path"=w1553) -> ("error out"=w1550:errorcluster, "Limits"=w1544:T25[], "File Version"=w1551:string, "File Name"=w1552:string, "Limits in Variant"=w1549:variant, "FaultCode Prefix"=w1542:i32)  [unwired: 4 in]
            n770 = case shown="No Error" w1550 {
              selector: w1550 -> [w1598 w1601]
              tunnel: w1546 -> [w1600 w1602]
              tunnel: [w1599 w1602] -> w1554
              tunnel: [w1598 w1601] -> w1545
              tunnel: w1549 -> [w1597 _]
              tunnel: w1551 -> [w1588 _]
              tunnel: w1552 -> [w1586 _]
              tunnel: w1548 -> [w1591 _]
              tunnel: w1544 -> [w1589 _]
              tunnel: w1542 -> [w1585 _]
              frame No Error {
                n771 = call <vilib>:"File.Remove Name Extension.vi"("File Name"=w1586) -> ("Name Less Ext"=w1587:string)  [unwired: 1 in, 1 out]
                n772 = Bundle By Name(cluster=T31 {"Name"="", "PN"="", "Version"="", "Note"=""} ("Software Items"), "Name"=w1587, "PN"="" ("Name"), "Version"=w1588, "Note"=w1586) -> (w1596:T31)
                n773 = Bundle By Name(cluster=w1600, "Lists.FaultPrefix"=w1585, "Lists.Limit File"=w1586, "Lists.Limit Ver"=w1588, "Lists.Limits"=w1597) -> (w1599:T73)
                n774 = Build Array(w1596) -> (w1595:T31[])
                n775 = To Variant(anything=w1595) -> (Variant=w1594:variant)
                n776 = call <vilib>:"Q.Enqueue Task.vi"("Data1"=w1594, "Task Name"="Client - SW Items", "Q In"=w1591) -> ()  [unwired: 7 in, 2 out]
                "Limits" <- w1589
                "Limit File Name" <- w1586
                "Limit File Ver" <- w1588
              }
              frame Error {
              }
            }
          }
          frame "Read Limits from Oper File" {
            n777 = Unbundle By Name(w1608) -> ("Cfg.Dirs.Config"=w1610:path)
            n778 = Build Path(base path=w1610, name or relative path="Limits") -> (appended path=w1607:path)
            n779 = call "File Dialog"("start path"=w1607, "prompt"="Select Limit File", "pattern (all files)"="*.xml") -> ("selected path"=w1604:path, "cancelled"=w1603:bool)  [unwired: 9 in, 2 out]
            n780 = case shown="True" w1603 {
              tunnel: [w1624 w1642] -> w1614
              tunnel: w1613 -> [w1619 _]
              tunnel: w1612 -> [w1618 w1642]
              tunnel: [w1617 _] -> w1611
              tunnel: w1604 -> [w1615 _]
              frame False {
                n781 = call "Result.Load Test Limits from XML File.vi"("Limit File Path"=w1615) -> ("error out"=w1621:errorcluster, "Limits"=w1616:T25[], "File Version"=w1622:string, "File Name"=w1623:string, "Limits in Variant"=w1620:variant)  [unwired: 5 in, 1 out]
                n782 = case shown="No Error" w1621 {
                  selector: w1621 -> [w1637 w1640]
                  tunnel: w1618 -> [w1639 w1641]
                  tunnel: [w1638 w1641] -> w1624
                  tunnel: [w1637 w1640] -> w1617
                  tunnel: w1620 -> [w1636 _]
                  tunnel: w1622 -> [w1625 _]
                  tunnel: w1623 -> [w1626 _]
                  tunnel: w1619 -> [w1629 _]
                  tunnel: w1616 -> [w1627 _]
                  frame No Error {
                    n783 = local write "Limits"(w1627) -> ()
                    n784 = Bundle By Name(cluster=T31 {"Name"="", "PN"="", "Version"="", "Note"=""} ("Software Items"), "Name"="Test Limits", "PN"="" ("Name"), "Version"=w1625, "Note"=w1626) -> (w1635:T31)
                    n785 = Bundle By Name(cluster=w1639, "Lists.Limit File"=w1626, "Lists.Limit Ver"=w1625, "Lists.Limits"=w1636) -> (w1638:T73)
                    n786 = local write "Limit File Name"(w1626) -> ()
                    n787 = local write "Limit File Ver"(w1625) -> ()
                    n788 = Build Array(w1635) -> (w1634:T31[])
                    n789 = To Variant(anything=w1634) -> (Variant=w1633:variant)
                    n790 = call <vilib>:"Q.Enqueue Task.vi"("Data1"=w1633, "Task Name"="Client - SW Items", "Q In"=w1629) -> ()  [unwired: 7 in, 2 out]
                  }
                  frame Error {
                  }
                }
              }
              frame True {
              }
            }
          }
          frame "Repeat Kill" {
            n791 = call <vilib>:"Scheduler.Delete Task.vi"("Sched Name"="Repeat Notification", "Q In"=w1651) -> ("Q Out"=w1647:refnum<queue>)  [unwired: 8 in, 1 out]
            n792 = call <vilib>:"Scheduler.Delete Task.vi"("Sched Name"="Repeat Sequence", "Q In"=w1647) -> ("Q Out"=w1648:refnum<queue>)  [unwired: 8 in, 1 out]
            n793 = call <vilib>:"Scheduler.Delete Task.vi"("Sched Name"="Repeat Sequence - Auto", "Q In"=w1648) -> ()  [unwired: 8 in, 2 out]
            n794 = Bundle By Name(cluster=w1654, "Repeat(s)"=-1.0) -> (w1653:T73)
            n795 = property on="Repeat Notificaiton" class="Str"("Visible"=FALSE) -> ()  [unwired: 2 in, 2 out]
            n796 = local write "Repeat Seq"(FALSE ("Repeat Seq")) -> ()
            n797 = property on="Kill AutoLnch" class="Bool"("Visible"=FALSE) -> ()  [unwired: 2 in, 2 out]
          }
          frame "Repeat Notification" {
            w1660 = "Repeat Notification"
            n798 = Unbundle By Name(w1664) -> ("Repeat(s)"=w1663:dbl)
            n799 = local read "End Time"() -> (w1657:timestamp)
            n800 = call <vilib>:"Scheduler.AddTask.vi"("Interval(s)"=0.5, "Task Name"=w1660, "Sched Name"=w1660, "Q In"=w1661) -> ()  [unwired: 6 in, 2 out]
            n801 = Get Date/Time In Seconds() -> (seconds since 1Jan1904=w1658:timestamp)
            n802 = Subtract(x=w1658, y=w1657) -> (x-y=w1656:dbl)
            n803 = Subtract(x=w1663, y=w1656) -> (x-y=w1662:dbl)
            n804 = Format Into String(format string="Seq auto launch in %.2f s.", w1662) -> (resulting string=→"Repeat Notificaiton":string)  [unwired: 2 in, 1 out]
          }
